vi "Pointer.Read (Boolean).vi"(8 "error in (no error)":errorcluster, 11 "pointer in":u64) -> (0 "error out":errorcluster, 2 "value":bool, 3 "pointer out":u64)   [LabVIEW 2016, in "VeriStand Data.lvlib"]
doc: "Read a value from the provided <B>pointer</B>."
uses:
  VeriStand Data.lvlib
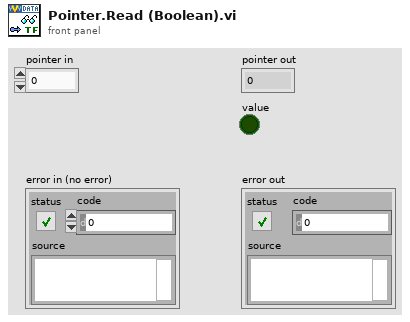
[diagram p1: front panel]
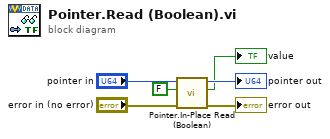
[diagram p0: block diagram]
diagram:
  n1 = call "Pointer.In-Place Read (Boolean).vi"("error in (no error)"="error in (no error)", "value in"=FALSE, "pointer in"="pointer in") -> ("error out"=→"error out":errorcluster, "value out"=→"value":bool, "pointer out"=→"pointer out":u64)  [unwired: 6 in]
